vi "数据查询_仪器数据.vi"() -> ()   [LabVIEW 2016]
uses:
  <vilib>/Utility/miscctls.llb/LVRowAndColumnUnsignedTypeDef.ctl
  <vilib>/Utility/miscctls.llb/LVPointTypeDef.ctl
panel:
  in  "工作模式":string(combo)="全部数据"
  in  "查询":bool
  in  "结束日期":string="2020/01/01"
  in  "起始日期":string="2010/01/01"
  in  "组合框":string(combo)
  out "数据表":string[][](table)
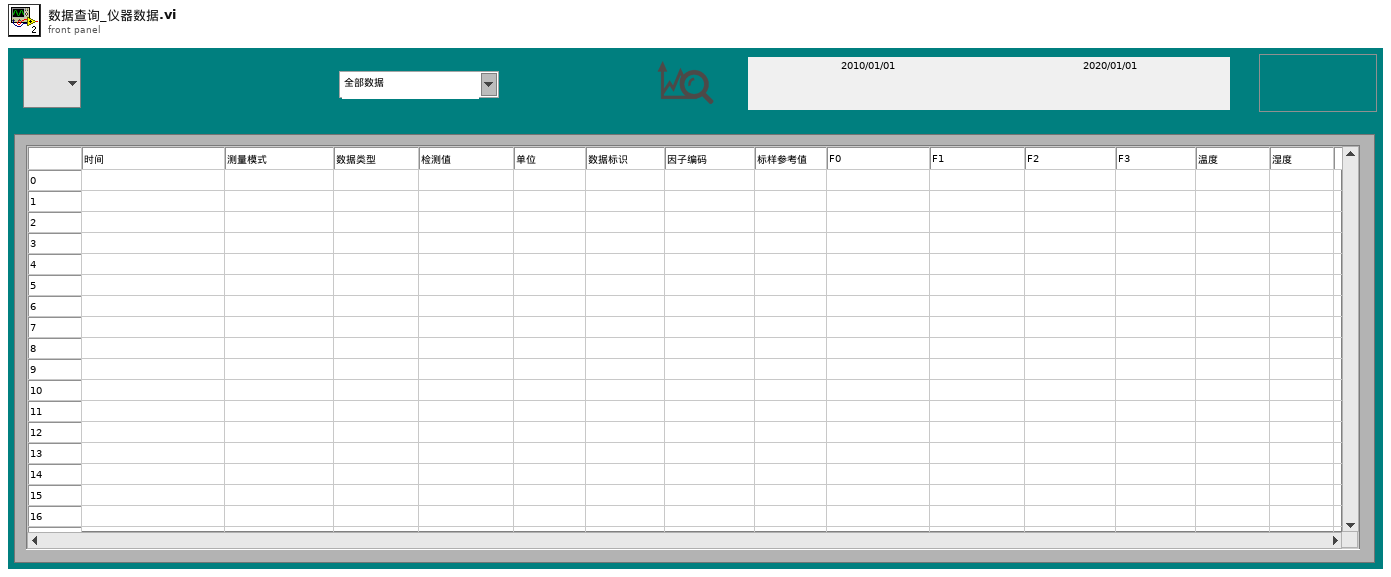
[diagram p1: front panel]
types:
  T1 = typedef "LVRowAndColumnUnsignedTypeDef.ctl" = cluster{"Row":u32, "Column":u32}
  T2 = typedef "LVPointTypeDef.ctl" = cluster{"Horizontal":i16, "Vertical":i16}
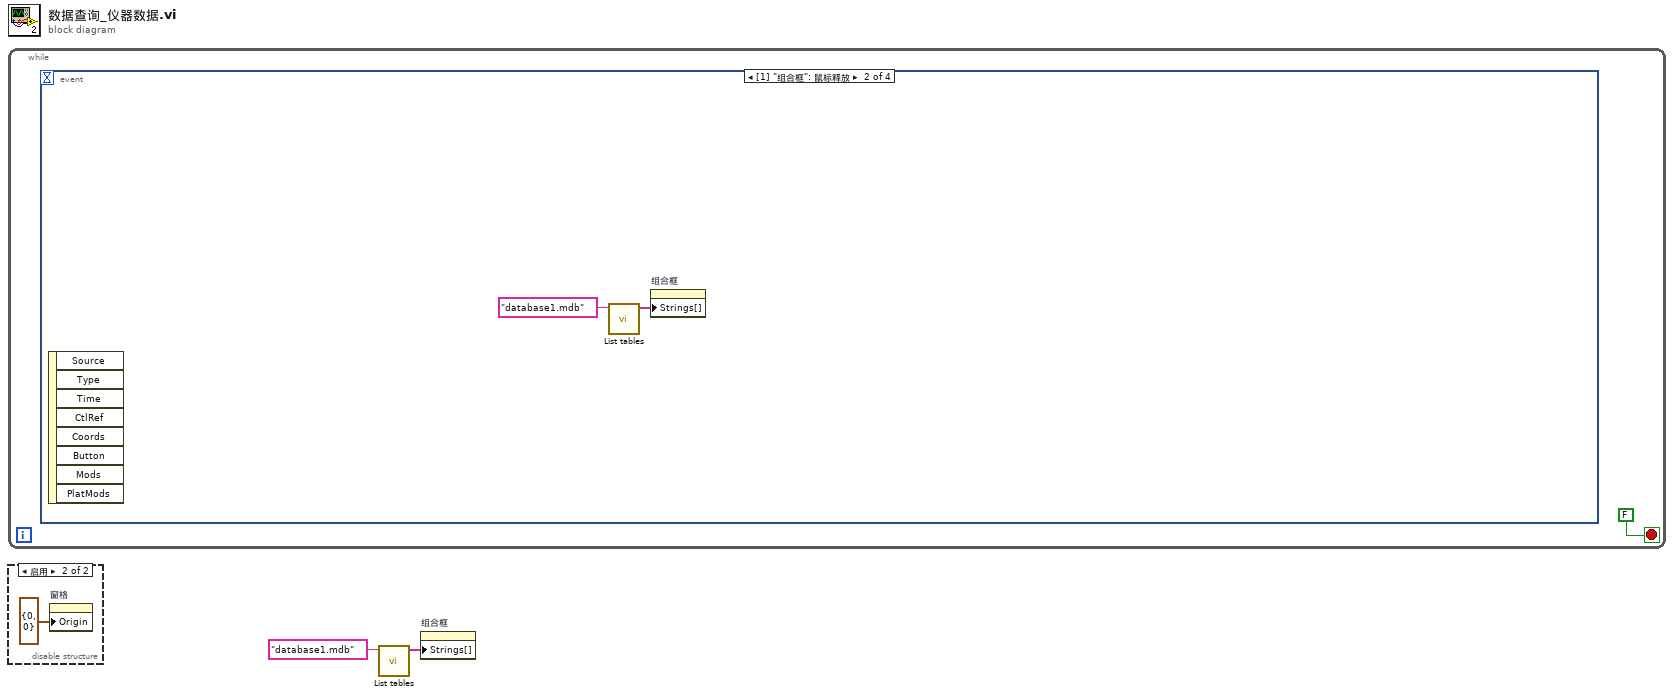
[diagram p0: block diagram]
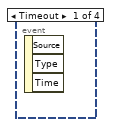
[diagram p2: hidden frame]
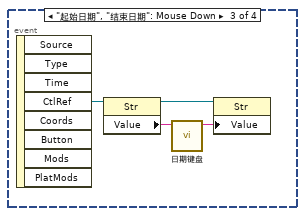
[diagram p3: hidden frame]
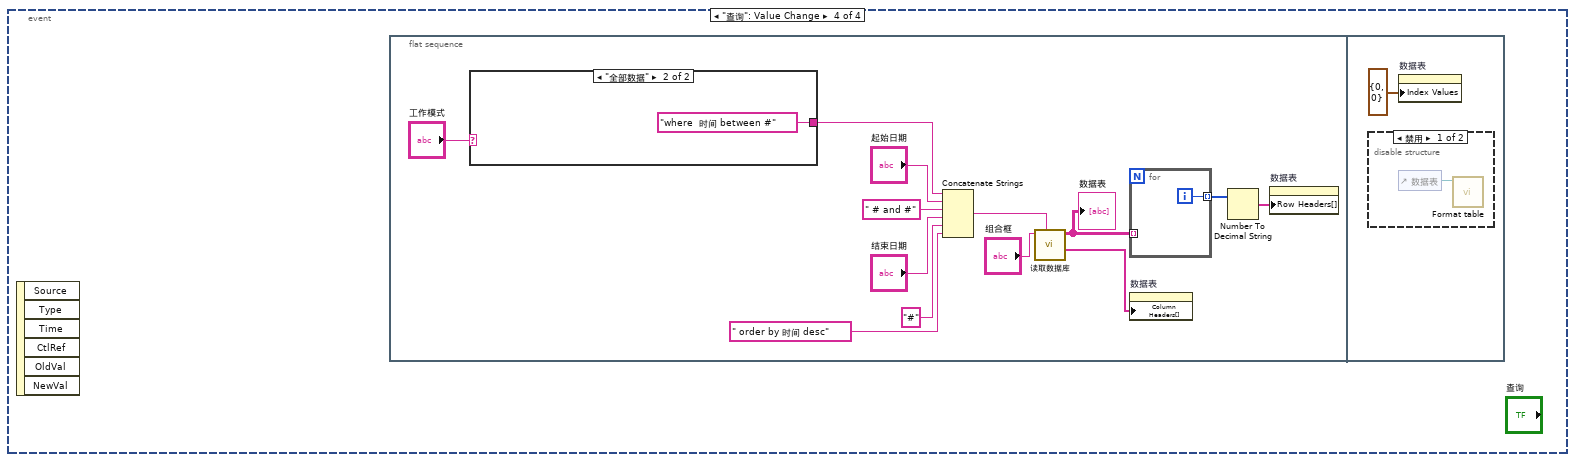
[diagram p4: hidden frame]
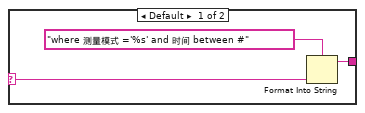
[diagram p5: hidden frame]
diagram:
  n1 = while {
    stop <- FALSE stop-if-true
    n2 = event shown="[1] \"组合框\": 鼠标释放" {
      selector: _ -> [_ _ _ _]
      dyn-events: _ -> [_ _ _ _]
      timeout: _ -> [_ _ _ _]
      event Timeout {
        n3 = event-data() -> ()  [unwired: 1 in, 3 out]
      }
      event "组合框": Mouse Up {
        n4 = event-data() -> ()  [unwired: 1 in, 8 out]
        n5 = call "List tables.vi"("database"="database1.mdb") -> ("tables"=w5:string[])  [unwired: 9 in, 1 out]
        n6 = property on="组合框" class="CmbBox"("Strings[]"=w5) -> ()  [unwired: 2 in, 2 out]
      }
      event "起始日期", "结束日期": Mouse Down {
        n7 = event-data() -> ("CtlRef"=w9:refnum<vi>)  [unwired: 1 in, 7 out]
        n8 = property class="Str"(reference=w9) -> (reference out=w7:refnum<vi>, "Value"=w8:string)  [unwired: 1 in, 1 out]
        n9 = call "日期键盘.vi"("原值"=w8) -> ("x+y"=w6:string)  [unwired: 10 in]
        n10 = property class="Str"(reference=w7, "Value"=w6) -> ()  [unwired: 1 in, 2 out]
      }
      event "查询": Value Change {
        n11 = event-data() -> ()  [unwired: 1 in, 6 out]
        n12 = flat-sequence {
          frame #0 {
            n13 = case shown="\"全部数据\"" "工作模式" {
              selector: "工作模式" -> [w25 _]
              tunnel: [w23 "where  时间 between #" ("condition")] -> w10
              frame Default {
                n14 = Format Into String(format string="where 测量模式 ='%s' and 时间 between #" ("condition"), w25) -> (resulting string=w23:string)  [unwired: 2 in, 1 out]
              }
              frame "全部数据" {
              }
            }
            n15 = Concatenate Strings(w10, "起始日期", " # and #" ("condition"), "结束日期", "#" ("condition"), " order by 时间 desc" ("字符串")) -> (w21:string)
            n16 = call "读取数据库.vi"("condition"=w21, "组合框"="组合框") -> ("columns"=w17:string[], "表格"=w14:string[][])  [unwired: 6 in, 2 out]
            "数据表" <- w14
            n17 = for {
              tunnel: w14 -> [_] mode=indexing
              tunnel: [w27] -> w13 mode=indexing
              i -> [w27]
            }
            n18 = property on="数据表" class="Tbl (严格)"("Column Headers[]"=w17) -> ()  [unwired: 2 in, 2 out]
            n19 = Number To Decimal String(number=w13) -> (decimal integer string=w12:string[])  [unwired: 1 in]
            n20 = property on="数据表" class="Tbl (严格)"("Row Headers[]"=w12) -> ()  [unwired: 2 in, 2 out]
          }
          frame #1 {
            n21 = disable-structure shown="禁用" {
              frame Disabled {
                n22 = control-ref of="数据表"() -> (w29:refnum<vi>)
                n23 = call "Format table.vi"("Table输入"=w29) -> ()  [unwired: 11 in]
              }
              frame Enabled {
              }
            }
            n24 = property on="数据表" class="Tbl (严格)"("Index Values"=T1 {"Row"=0, "Column"=0} ("索引值")) -> ()  [unwired: 2 in, 2 out]
          }
        }
      }
    }
  }
  n25 = disable-structure shown="启用" {
    frame Disabled {
    }
    frame Enabled {
      n26 = property on="窗格" class="Pane"("Origin"=T2 {"Horizontal"=0, "Vertical"=0} ("原点")) -> ()  [unwired: 2 in, 2 out]
    }
  }
  n27 = call "List tables.vi"("database"="database1.mdb") -> ("tables"=w1:string[])  [unwired: 9 in, 1 out]
  n28 = property on="组合框" class="CmbBox"("Strings[]"=w1) -> ()  [unwired: 2 in, 2 out]
